vi "Positions in Use.vi"(0 "Sytem #":u8=1 min=1 max=16, 1 "AutoAge.ini  File Path":path=path "\\\\Beco\\autoage/config/autoage.ini", 4 "Oscillator Type":string) -> (2 "Positions In Use":i32, 3 "Total Positions":i32)   [LabVIEW 2021]
uses:
  Main Controls System v8.0/AutoAge Globals.vi
panel:
  out "?":string
  # "Display Rack Information & Cross Reference"
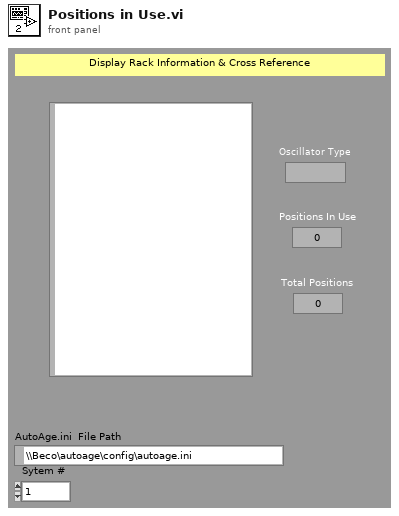
[diagram p1: front panel]
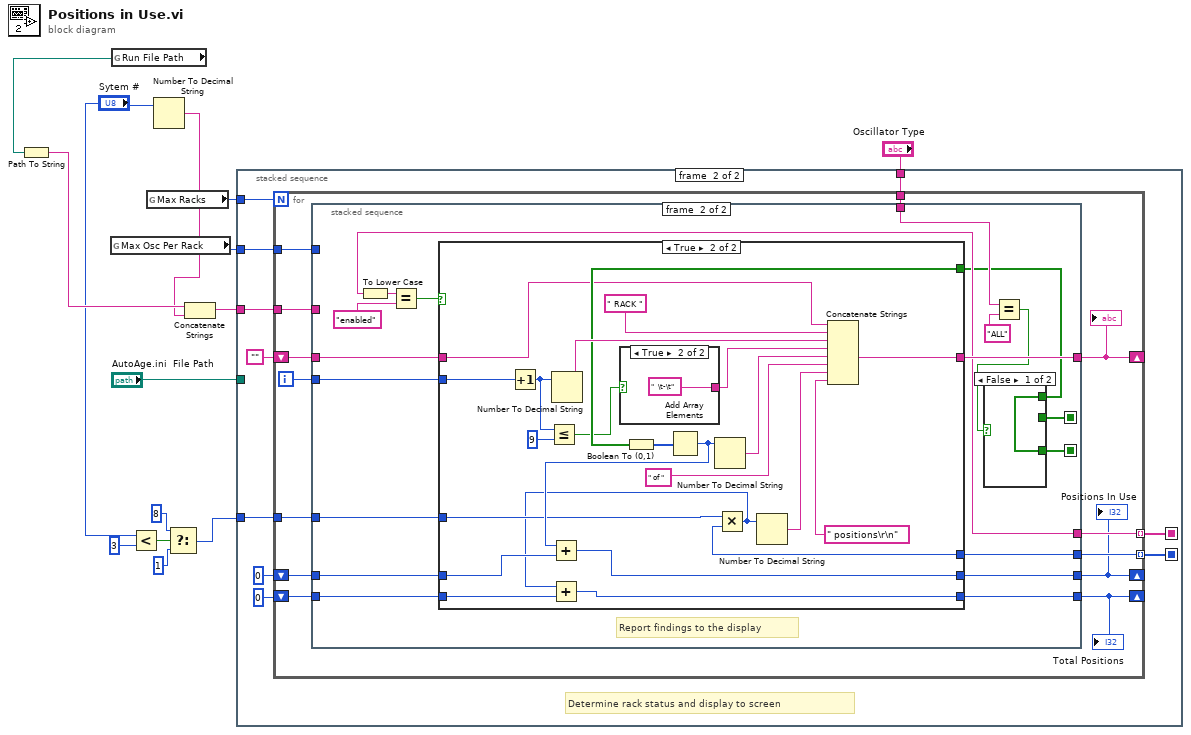
[diagram p0: block diagram]
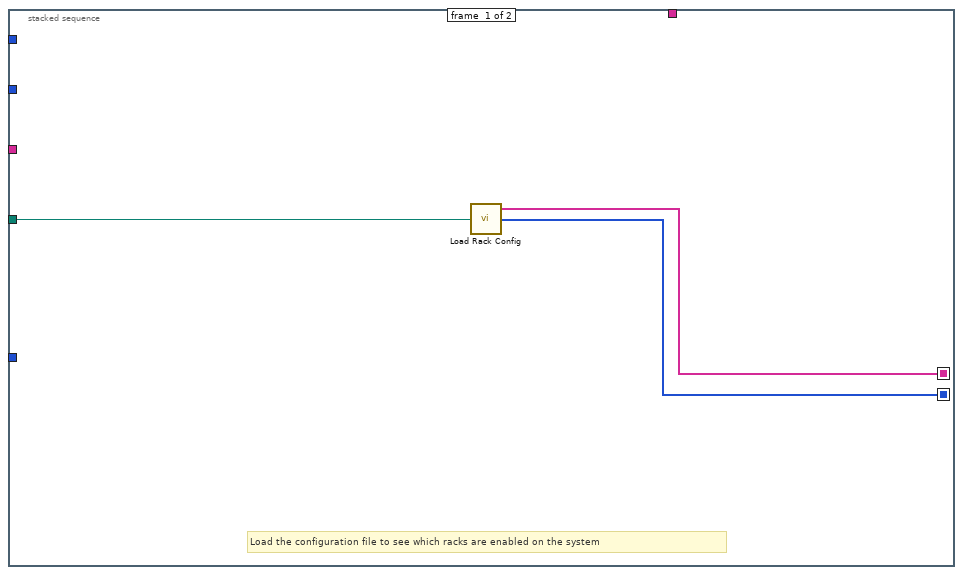
[diagram p2: hidden frame]
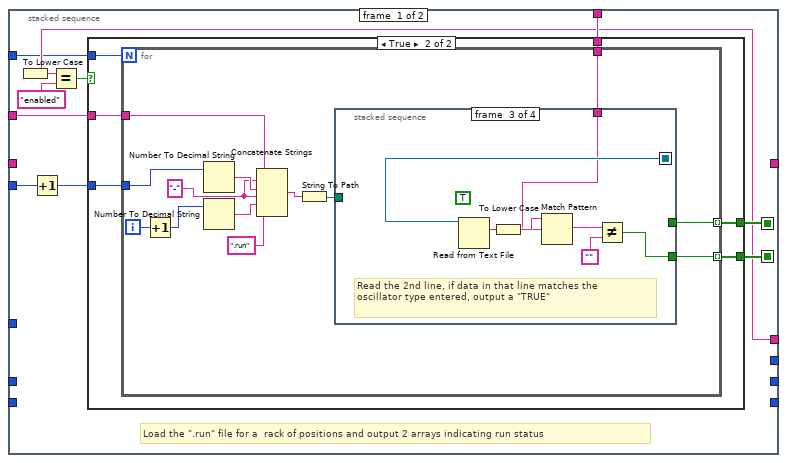
[diagram p3: hidden frame]
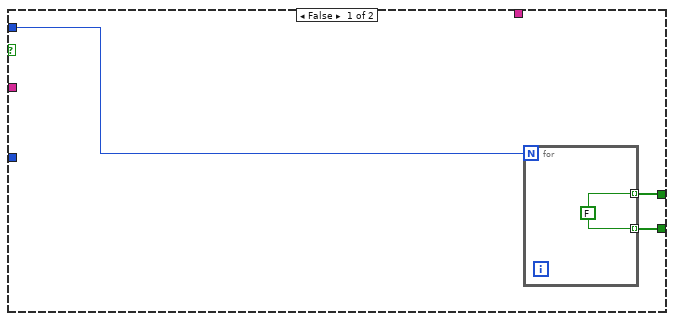
[diagram p4: hidden frame]
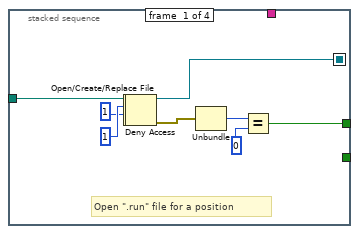
[diagram p5: hidden frame]
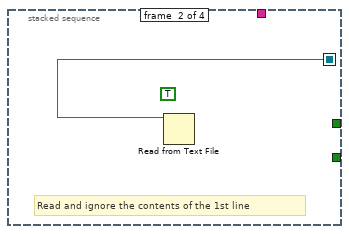
[diagram p6: hidden frame]
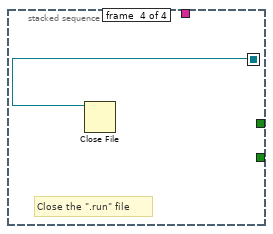
[diagram p7: hidden frame]
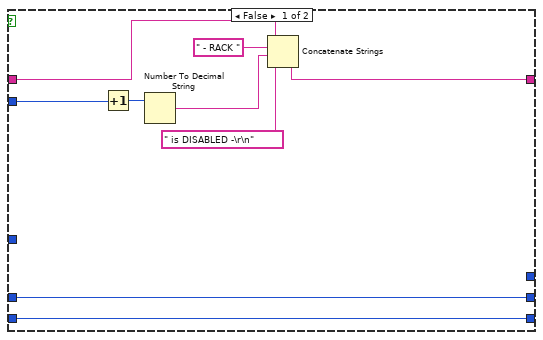
[diagram p9: hidden frame]
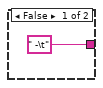
[diagram p10: hidden frame]
diagram:
  n1 = global read "AutoAge Globals.vi" "Max Osc Per Rack"() -> (w7:u16)
  n2 = global read "AutoAge Globals.vi" "Run File Path"() -> (w12:path)
  n3 = Path To String(path=w12) -> (string=w10:string)
  n4 = Less?(x="Sytem #", y=u8 3) -> (x < y?=w4:bool)
  n5 = global read "AutoAge Globals.vi" "Max Racks"() -> (w8:u8)
  n6 = Number To Decimal String(number="Sytem #") -> (decimal integer string=w9:string)  [unwired: 1 in]
  n7 = Select(t=u8 8, s=w4, f=u8 1) -> (s? t:f=w1:u8)
  n8 = Concatenate Strings(w10, w9) -> (w11:string)
  n9 = stacked-sequence {
    seq-local: [w17 _] -> [_ w27]
    seq-local: [w16 _] -> [_ w23]
    tunnel: "Oscillator Type" -> [_ w22]
    tunnel: "AutoAge.ini  File Path" -> [w15 _]
    tunnel: w11 -> [_ w21]
    tunnel: w8 -> [_ w20]
    tunnel: w7 -> [_ w19]
    tunnel: w1 -> [_ w18]
    frame #0 {
      # "Load the configuration file to see which racks are enabled on the system"
      n10 = call "Load Rack Config"("AutoAge.ini  File Path"=w15) -> ("Rack Status"=w16:string[], "# of Cards"=w17:i32[])  [unwired: 1 out]
    }
    frame #1 {
      # "Determine rack status and display to screen"
      n11 = for {
        N: w20 -> [_]
        tunnel: w27 -> [w39] mode=indexing
        shift-right: [w34] -> _
        shift-left: "" -> [w38]
        shift-right: [w31] -> _
        shift-left: 0 -> [w36]
        shift-right: [w32] -> _
        shift-left: 0 -> [w35]
        tunnel: w23 -> [w37] mode=indexing
        tunnel: w22 -> [w33]
        tunnel: w21 -> [w30]
        tunnel: w19 -> [w29]
        tunnel: w18 -> [w28]
        i -> [w40]
        n12 = stacked-sequence {
          seq-local: [w50 _] -> [_ w97]
          seq-local: [w49 _] -> [_ w96]
          tunnel: w40 -> [w51 w112]
          tunnel: w39 -> [_ w110]
          tunnel: [_ w111] -> w34
          tunnel: w38 -> [_ w109]
          tunnel: w37 -> [w45 w106]
          tunnel: w36 -> [_ w104]
          tunnel: w35 -> [_ w103]
          tunnel: [_ w102] -> w31
          tunnel: [_ w101] -> w32
          tunnel: w33 -> [w48 w100]
          tunnel: w30 -> [w42 _]
          tunnel: w29 -> [w41 _]
          tunnel: w28 -> [_ w94]
          frame #0 {
            # "Load the \".run\" file for a  rack of positions and output 2 arrays indicating run status"
            n13 = To Lower Case(string=w45) -> (all lower case string=w46:string)
            n14 = Increment(x=w51) -> (x+1=w43:i32)
            n15 = Equal?(x=w46, y="enabled") -> (x = y?=w44:bool)
            n16 = case shown="True" w44 {
              tunnel: w43 -> [_ w61]
              tunnel: [w54 w60] -> w50
              tunnel: [w53 w59] -> w49
              tunnel: w48 -> [_ w58]
              tunnel: w42 -> [_ w57]
              tunnel: w41 -> [w52 w56]
              frame False {
                n17 = for {
                  N: w52 -> [_]
                  tunnel: [w55] -> w54 mode=indexing
                  tunnel: [w55] -> w53 mode=indexing
                  w55 = FALSE
                }
              }
              frame True {
                n18 = for {
                  N: w56 -> [_]
                  tunnel: w61 -> [w65]
                  tunnel: [w72] -> w60 mode=indexing
                  tunnel: [w71] -> w59 mode=indexing
                  tunnel: w58 -> [w70]
                  tunnel: w57 -> [w62]
                  i -> [w73]
                  w63 = "-"
                  n19 = Increment(x=w73) -> (x+1=w66:i32)
                  n20 = Number To Decimal String(number=w65) -> (decimal integer string=w69:string)  [unwired: 1 in]
                  n21 = Number To Decimal String(number=w66) -> (decimal integer string=w68:string)  [unwired: 1 in]
                  n22 = Concatenate Strings(w62, w63, w69, w63, w68, ".run") -> (w64:string)
                  n23 = String To Path(string=w64) -> (path=w74:path)
                  n24 = stacked-sequence {
                    seq-local: [w78 _ _ _] -> [_ w85 w92 w93]
                    tunnel: [w77 _ _ _] -> w72
                    tunnel: w74 -> [w84 _ _ _]
                    tunnel: [_ _ w87 _] -> w71
                    tunnel: w70 -> [_ _ w86 _]
                    frame #0 {
                      # "Open \".run\" file for a position"
                      n25 = Open/Create/Replace File(file path (use dialog)=w84, access (0:read/write)=1) -> (refnum out=w75:refnum<file>, error out=w76:errorcluster)  [unwired: 4 in, 1 out]
                      n26 = Deny Access(4:w76, 6:1, 7:w75) -> (0:w81:errorcluster, 3:w78:refnum<file>)
                      n27 = Unbundle(w81) -> ("code"=w79:i32)  [unwired: 2 out]
                      n28 = Equal?(x=w79, y=0) -> (x = y?=w77:bool)
                    }
                    frame #1 {
                      (unwired) TRUE
                      # "Read and ignore the contents of the 1st line"
                      n29 = Read from Text File(file (use dialog)=w85) -> ()  [unwired: 3 in, 4 out]
                    }
                    frame #2 {
                      (unwired) TRUE
                      # "Read the 2nd line, if data in that line matches the\noscillator type entered, output a \"TRUE\""
                      n30 = Read from Text File(file (use dialog)=w92) -> (text=w91:string)  [unwired: 3 in, 3 out]
                      n31 = To Lower Case(string=w91) -> (all lower case string=w90:string)
                      n32 = Match Pattern(string=w90, regular expression=w86) -> (match substring=w89:string)  [unwired: 1 in, 3 out]
                      n33 = Not Equal?(x=w89, y="") -> (x != y?=w87:bool)
                    }
                    frame #3 {
                      # "Close the \".run\" file"
                      n34 = Close File(refnum=w93) -> ()  [unwired: 1 in, 2 out]
                    }
                  }
                }
              }
            }
          }
          frame #1 {
            # "Report findings to the display"
            n35 = To Lower Case(string=w106) -> (all lower case string=w107:string)
            n36 = Equal?(x=w107, y="enabled") -> (x = y?=w105:bool)
            n37 = Equal?(x=w100, y="ALL") -> (x = y?=w98:bool)
            n38 = case shown="False" w98 {
              tunnel: w97 -> [_ w114]
              tunnel: w96 -> [w113 _]
              tunnel: [w113 w114] -> w95
              frame False {
              }
              frame True {
              }
            }
            n39 = case shown="True" w105 {
              tunnel: w112 -> [w120 w146]
              tunnel: [w115 w124] -> w111
              tunnel: w95 -> [_ w143]
              tunnel: w110 -> [_ w129]
              tunnel: w109 -> [w118 w137]
              tunnel: w104 -> [w123 w132]
              tunnel: w103 -> [w122 w130]
              tunnel: [w123 w126] -> w102
              tunnel: [w122 w125] -> w101
              tunnel: w94 -> [_ w128]
              frame False {
                n40 = Increment(x=w120) -> (x+1=w121:i32)
                n41 = Number To Decimal String(number=w121) -> (decimal integer string=w119:string)  [unwired: 1 in]
                n42 = Concatenate Strings(w118, " - RACK ", w119, " is DISABLED -\r\n") -> (w115:string)
              }
              frame True {
                n43 = Increment(x=w146) -> (x+1=w135:i32)
                n44 = Less Or Equal?(x=w135, y=9) -> (x <= y?=w133:bool)
                n45 = Number To Decimal String(number=w135) -> (decimal integer string=w145:string)  [unwired: 1 in]
                n46 = case shown="True" w133 {
                  tunnel: [" -\t" "  \t-\t"] -> w136
                  frame False {
                  }
                  frame True {
                  }
                }
                n47 = Boolean To (0,1)(Boolean=w143) -> (0, 1=w142:i16[])
                n48 = Add Array Elements(numeric array=w142) -> (sum=w131:i16)
                n49 = Add(x=w131, y=w132) -> (x+y=w126:i32)
                n50 = Number To Decimal String(number=w131) -> (decimal integer string=w141:string)  [unwired: 1 in]
                n51 = Multiply(x=w128, y=w129) -> (x*y=w127:i32)
                n52 = Add(x=w127, y=w130) -> (x+y=w125:i32)
                n53 = Number To Decimal String(number=w127) -> (decimal integer string=w139:string)  [unwired: 1 in]
                n54 = Concatenate Strings(w137, " RACK ", w145, w136, w141, " of ", w139, " positions\r\n") -> (w124:string)
              }
            }
          }
        }
        "Total Positions" <- w32
        "Positions In Use" <- w31
        "?" <- w34
      }
    }
  }
